vi "_New SequenceFile.vi"(8 "error in (no error)":errorcluster, 11 "Engine in":refnum<class "Engine.lvclass">) -> (0 "error out":errorcluster, 2 "New SequenceFile":refnum<class "SequenceFile.lvclass">, 3 "Engine out":refnum<class "Engine.lvclass">)   [LabVIEW 2020, in "TSnax.lvlib" / "Engine.lvclass"]
uses:
  Engine.lvclass
  Engine.lvclass/Engine.ctl
  SequenceFile/SequenceFile.lvclass
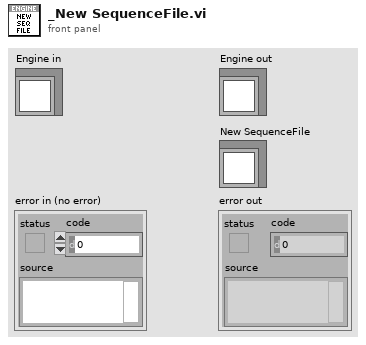
[diagram p1: front panel]
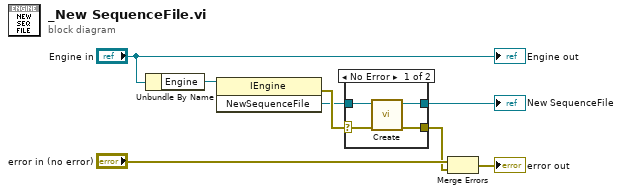
[diagram p0: block diagram]
diagram:
  n1 = Unbundle By Name("Engine in") -> ("Engine"=w6:refnum<k7>)
  n2 = invoke class="IEngine" method="NewSequenceFile"(reference=w6) -> (error out=w8:errorcluster, "NewSequenceFile"=w5:refnum<k7>)  [unwired: 2 in, 1 out]
  n3 = case shown="No Error" w8 {
    selector: w8 -> [w12 w13]
    tunnel: w5 -> [w11 _]
    tunnel: [w9 w13] -> w3
    tunnel: [w10 _] -> w1
    frame No Error {
      n4 = call "Create.vi"("error in (no error)"=w12, "SequenceFile"=w11) -> ("error out"=w9:errorcluster, "SequenceFile out"=w10:refnum<class "SequenceFile.lvclass">)  [unwired: 8 in]
    }
    frame Error {
    }
  }
  "New SequenceFile" <- w1
  n5 = Merge Errors("error in (no error)", w3) -> (→"error out":errorcluster)
  "Engine out" <- "Engine in"
